vi "Sweep Control Loop.vi"(8 "error in (no error)":errorcluster, 11 "SweepControl in":refnum<class "SweepControl.lvclass">) -> ()   [LabVIEW 2019, in "SweepControl.lvclass"]
uses:
  <userlib>/LevyLab/Transport/SweepControl/SweepControl.lvclass
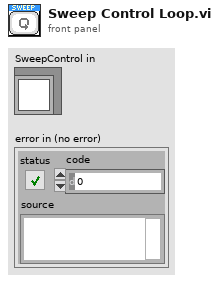
[diagram p1: front panel]
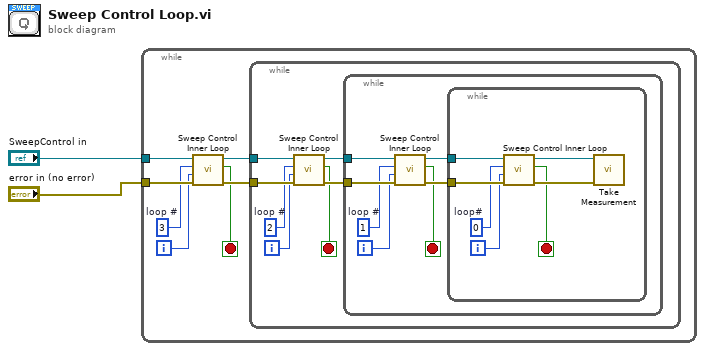
[diagram p0: block diagram]
diagram:
  n1 = while {
    tunnel: "error in (no error)" -> [w7]
    tunnel: "SweepControl in" -> [w9]
    i -> [w4]
    stop <- w3 stop-if-true
    w5 = 3  # loop #
    n2 = call <userlib>:"Sweep Control Inner Loop.vi"("error in (no error)"=w7, "inner loop index"=w4, "loop #"=w5, "SweepControl in"=w9) -> ("error out"=w6:errorcluster, "Stop?"=w3:bool, "SweepControl out"=w8:refnum<class "SweepControl.lvclass">)  [unwired: 5 in]
    n3 = while {
      tunnel: w6 -> [w15]
      tunnel: w8 -> [w16]
      i -> [w11]
      stop <- w10 stop-if-true
      w14 = 2  # loop #
      n4 = call <userlib>:"Sweep Control Inner Loop.vi"("error in (no error)"=w15, "inner loop index"=w11, "loop #"=w14, "SweepControl in"=w16) -> ("error out"=w13:errorcluster, "Stop?"=w10:bool, "SweepControl out"=w12:refnum<class "SweepControl.lvclass">)  [unwired: 5 in]
      n5 = while {
        tunnel: w13 -> [w23]
        tunnel: w12 -> [w22]
        i -> [w18]
        stop <- w17 stop-if-true
        w21 = 1  # loop #
        n6 = call <userlib>:"Sweep Control Inner Loop.vi"("error in (no error)"=w23, "inner loop index"=w18, "loop #"=w21, "SweepControl in"=w22) -> ("error out"=w20:errorcluster, "Stop?"=w17:bool, "SweepControl out"=w19:refnum<class "SweepControl.lvclass">)  [unwired: 5 in]
        n7 = while {
          tunnel: w20 -> [w30]
          tunnel: w19 -> [w26]
          i -> [w24]
          stop <- w25 stop-if-true
          w29 = 0  # loop#
          n8 = call <userlib>:"Sweep Control Inner Loop.vi"("error in (no error)"=w30, "inner loop index"=w24, "loop #"=w29, "SweepControl in"=w26) -> ("error out"=w28:errorcluster, "Stop?"=w25:bool, "SweepControl out"=w27:refnum<class "SweepControl.lvclass">)  [unwired: 5 in]
          n9 = call <userlib>:"Take Measurement.vi"("error in (no error)"=w28, "SweepControl in"=w27) -> ()  [unwired: 8 in, 2 out]
        }
      }
    }
  }
